vi "GetPrivateQueueConfig.vi"(8 "error in (no error)":errorcluster, 11 "DAQmx":refnum<class "DAQmx.lvclass">) -> (0 "error out":errorcluster, 3 "DAQmx out":refnum<class "DAQmx.lvclass">)   [LabVIEW 2019, in "DAQmx.lvclass"]
uses:
  DAQmx.lvclass
  DAQmx.lvclass/DAQmx.ctl
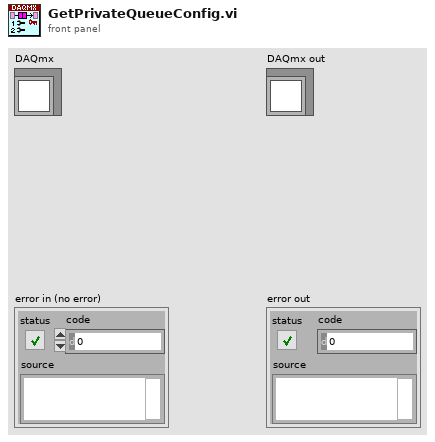
[diagram p1: front panel]
types:
  T1 = typedef "DAQmx.lvclass/DAQ.Config.Timing--Cluster.ctl" = cluster{"Sampling":T2, "sample mode":i32, "FsMode":T3, "Fs Multiplier":dbl, "Refresh Rate (Hz)":dbl, "Decimation.PreDSP":i32, "Decimation.PostDSP":i32, "Fs.Output":dbl}
  T2 = typedef "DAQmx.lvclass/DAQ.Config.Timing.Sampling--Cluster.ctl" = cluster{"Fs":dbl, "#s":i32}
  T3 = typedef "DAQmx.lvclass/DAQ.Config.Timing.Fs Mode--enum.ctl" = enum16{"Manual", "Auto Fs", "Max Fs"}
  T4 = typedef "DAQmx.lvclass/DAQ.Config.AO--Cluster--Array.ctl" = T5[]
  T5 = typedef "DAQmx.lvclass/DAQ.Config.AO--Cluster.ctl" = cluster{"Channels":tag, "Range":T6, "output terminal configuration":i32, "Type":T7}
  T6 = typedef "DAQmx.lvclass/DAQ.Config.AO.Range--enum.ctl" = enum16{"±0.1", "±1.0", "±10.0", ""}
  T7 = typedef "DAQmx.lvclass/DAQ.Config.Device Type--enum.ctl" = enum16{"None", "USB-4431", "PXI-446x"}
  T8 = typedef "DAQmx.lvclass/DAQ.Config.AI--Cluster--Array.ctl" = T9[]
  T9 = typedef "DAQmx.lvclass/DAQ.Config.AI--Cluster.ctl" = cluster{"Channels":tag, "Coupling":T10, "Range":T11, "input terminal configuration":i32, "Type":T7}
  T10 = typedef "DAQmx.lvclass/DAQ.Config.AI.Coupling--enum.ctl" = u16
  T11 = typedef "DAQmx.lvclass/DAQ.Config.AI.Range--enum.ctl" = enum16{"±0.316", "±1.00", "±3.16", "±10.0", "±31.6", "±42.4", ""}
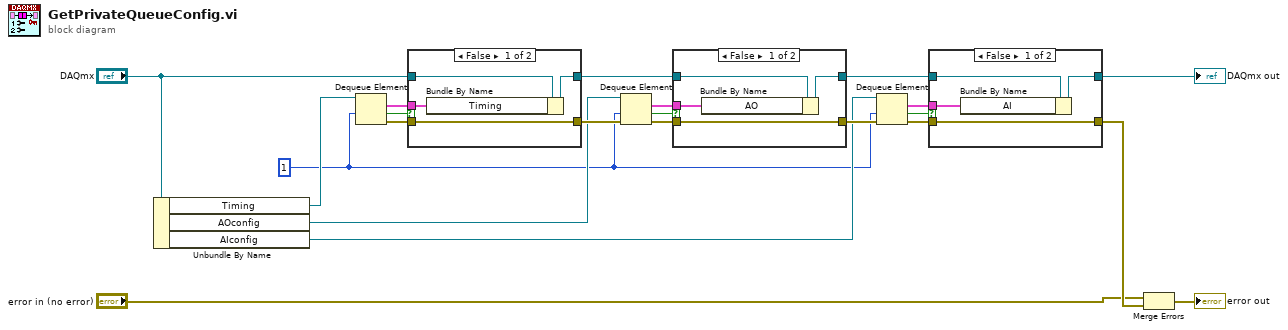
[diagram p0: block diagram]
diagram:
  w1 = 1 ("timeout in ms (-1)")
  n1 = Unbundle By Name("DAQmx") -> ("Timing"=w20:refnum<queue>, "AOconfig"=w8:refnum<queue>, "AIconfig"=w7:refnum<queue>)
  n2 = Dequeue Element(queue=w20, timeout in ms (-1)=w1) -> (element=w19:T1, timed out?=w18:bool, error out=w17:errorcluster)  [unwired: 1 in, 1 out]
  n3 = case shown="False" w18 {
    tunnel: "DAQmx" -> [w26 w27]
    tunnel: [w25 w27] -> w6
    tunnel: w19 -> [w24 _]
    tunnel: [w23 w28] -> w13
    tunnel: w17 -> [w23 w28]
    frame False {
      n4 = Bundle By Name(cluster=w26, "Timing"=w24) -> (w25:refnum<class "DAQmx.lvclass">)
    }
    frame True {
    }
  }
  n5 = Dequeue Element(queue=w8, timeout in ms (-1)=w1, error in (no error)=w13) -> (element=w14:T4, timed out?=w15:bool, error out=w16:errorcluster)  [unwired: 1 out]
  n6 = case shown="False" w15 {
    tunnel: w6 -> [w32 w33]
    tunnel: [w31 w33] -> w5
    tunnel: w14 -> [w30 _]
    tunnel: [w29 w34] -> w9
    tunnel: w16 -> [w29 w34]
    frame False {
      n7 = Bundle By Name(cluster=w32, "AO"=w30) -> (w31:refnum<class "DAQmx.lvclass">)
    }
    frame True {
    }
  }
  n8 = Dequeue Element(queue=w7, timeout in ms (-1)=w1, error in (no error)=w9) -> (element=w12:T8, timed out?=w11:bool, error out=w10:errorcluster)  [unwired: 1 out]
  n9 = case shown="False" w11 {
    tunnel: w5 -> [w38 w39]
    tunnel: [w37 w39] -> w21
    tunnel: w12 -> [w36 _]
    tunnel: [w35 w40] -> w4
    tunnel: w10 -> [w35 w40]
    frame False {
      n10 = Bundle By Name(cluster=w38, "AI"=w36) -> (w37:refnum<class "DAQmx.lvclass">)
    }
    frame True {
    }
  }
  "DAQmx out" <- w21
  n11 = Merge Errors("error in (no error)", w4) -> (→"error out":errorcluster)
